vi "CreateLeakagePowerVsTemperatureCurves.vi"() -> ()   [LabVIEW 2009]
uses:
  <instrlib>/BK Precision 91xx Series/BK Precision 91xx Series.lvlib
panel:
  out "error out":errorcluster
  in  "Serial Configuration":T1={"Parity(0:none)"=0, "Baud Rate (9600)"=9600, "Data Bits(8)"=8, "Flow Control(None)"=0, " Stop Bits(1.0)"=10} {"Stop Bits(1.0)" items=["1.0"=10, "1.5"=15, "2.0"=20]; "Flow Control(None)" items=["None", "XON/XOFF", "RTS/CTS", "XON/XOFF & RTS/CTS", "DTR/DSR", "XON/XOFF & DTR/DSR"]; "Data Bits(8)" items=["7"=7, "8"=8]; "Baud Rate (9600)" items=["2400"=2400, "4800"=4800, "9600"=9600, "19200"=19200, "38400"=38400]; "Parity(0:none)" items=["None", "Odd", "Even", "Mark", "Space"]}
  in  "VISA resource name":refnum<visa-resource-name>
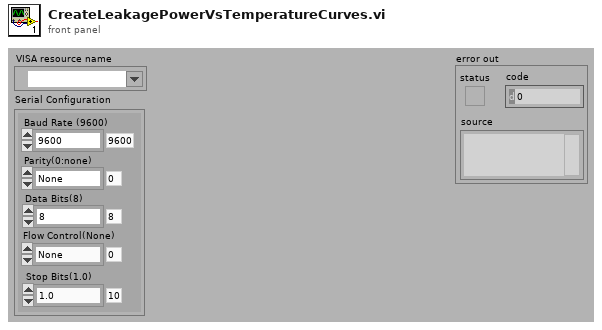
[diagram p1: front panel]
types:
  T1 = cluster{"Parity(0:none)":u16, "Baud Rate (9600)":u16, "Data Bits(8)":u16, "Flow Control(None)":u16, " Stop Bits(1.0)":u16}
  T2 = enum16{"open", "replace", "create", "open or create", "replace or create", "replace or create with confirmation"}
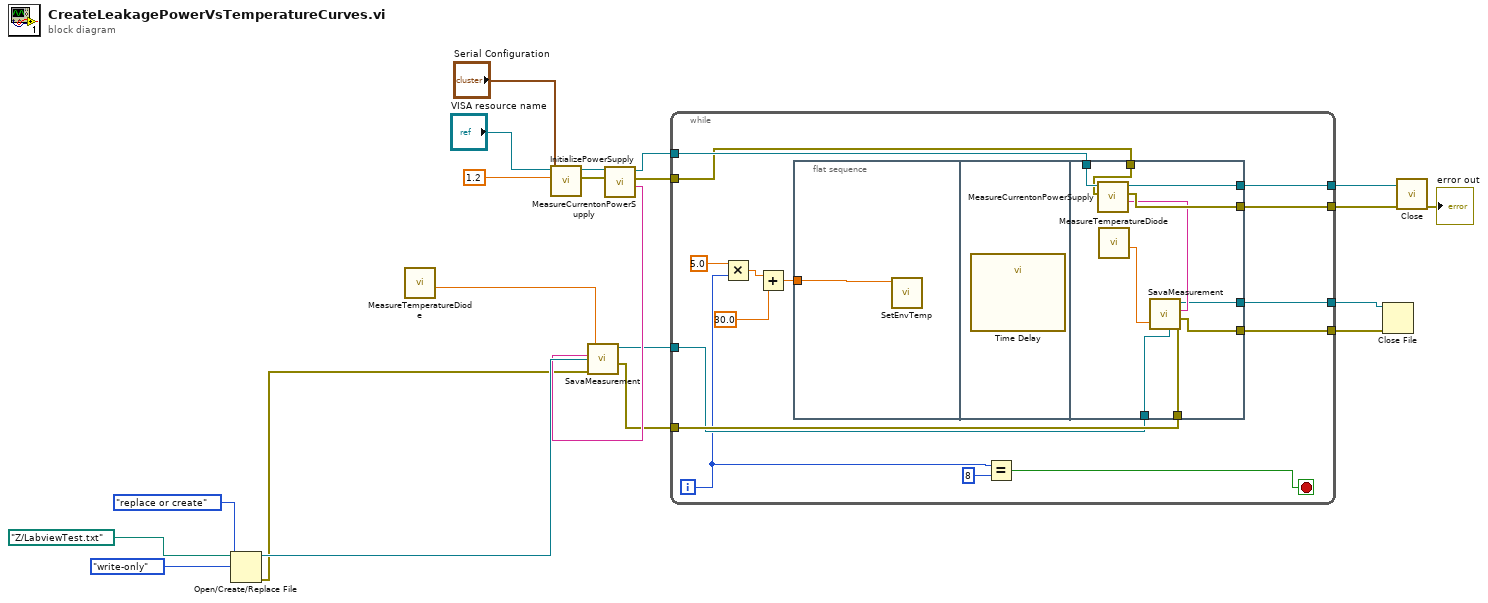
[diagram p0: block diagram]
diagram:
  n1 = Open/Create/Replace File(file path (use dialog)=path "Z:/LabviewTest.txt", operation (0:open)=T2."replace or create", access (0:read/write)=enum16{"read/write", "read-only", "write-only"}."write-only") -> (refnum out=w11:refnum<file>, error out=w6:errorcluster)  [unwired: 3 in, 1 out]
  n2 = call "MeasureTemperatureDiode.vi"() -> ("Celcius"=w5:dbl)  [unwired: 8 in, 3 out]
  n3 = call "InitializePowerSupply.vi"("Serial Configuration"="Serial Configuration", "Manual Range(0.00)"=1.2, "VISA resource name"="VISA resource name") -> ("error out"=w17:errorcluster, "VISA resource name out"=w18:refnum<visa-resource-name>)  [unwired: 7 in]
  n4 = call "MeasureCurrentonPowerSupply.vi"("error in (no error)"=w17, "VISA resource name"=w18) -> ("Measurement"=w7:string, "error out"=w15:errorcluster, "VISA resource name out"=w16:refnum<visa-resource-name>)  [unwired: 7 in]
  n5 = call "SavaMeasurement.vi"("error out"=w6, "Measurement"=w7, "refnum out"=w11, "DiodeTemperature"=w5) -> ("error out 2"=w4:errorcluster, "refnum out 2"=w3:refnum<file>)  [unwired: 1 in]
  n6 = while {
    tunnel: w16 -> [w32]
    tunnel: w15 -> [w31]
    tunnel: [w30] -> w14
    tunnel: [w29] -> w13
    tunnel: w4 -> [w28]
    tunnel: w3 -> [w27]
    tunnel: [w23] -> w2
    tunnel: [w22] -> w1
    i -> [w26]
    stop <- w24 stop-if-true
    n7 = Multiply(x=5.0 ("New temperature"), y=w26) -> (x*y=w34:dbl)
    n8 = Add(x=w34, y=30.0) -> (x+y=w33:dbl)
    n9 = flat-sequence {
      tunnel: w33 -> [w37]
      tunnel: w32 -> [w47]
      tunnel: w31 -> [w46]
      tunnel: [w45] -> w30
      tunnel: [w44] -> w29
      tunnel: w28 -> [w43]
      tunnel: w27 -> [w41]
      tunnel: [w39] -> w23
      tunnel: [w38] -> w22
      frame #0 {
        n10 = call "SetEnvTemp.vi"("New temperature"=w37) -> ()  [unwired: 10 in, 1 out]
      }
      frame #1 {
        n11 = call "Time Delay"() -> ()  [unwired: 11 in, 1 out]
      }
      frame #2 {
        n12 = call "MeasureCurrentonPowerSupply.vi"("error in (no error)"=w46, "VISA resource name"=w47) -> ("Measurement"=w40:string, "error out"=w44:errorcluster, "VISA resource name out"=w45:refnum<visa-resource-name>)  [unwired: 7 in]
        n13 = call "MeasureTemperatureDiode.vi"() -> ("Celcius"=w42:dbl)  [unwired: 8 in, 3 out]
        n14 = call "SavaMeasurement.vi"("error out"=w43, "Measurement"=w40, "refnum out"=w41, "DiodeTemperature"=w42) -> ("error out 2"=w39:errorcluster, "refnum out 2"=w38:refnum<file>)  [unwired: 1 in]
      }
    }
    n15 = Equal?(x=w26, y=8) -> (x = y?=w24:bool)
  }
  n16 = Close File(refnum=w1, error in=w2) -> ()  [unwired: 2 out]
  n17 = call <instrlib>:"Close.vi"("error in (no error)"=w13, "VISA resource name"=w14) -> ("error out"=→"error out":errorcluster)  [unwired: 9 in]
